vi "arduino_commands_subvi.vi"(0 "Shutter off":bool, 1 "Shutter on":bool, 2 "Go to step":bool, 3 "Constant speed":bool, 4 "Current Step":bool, 5 "Set zero":bool, 6 "wait until completion? (T)":bool=TRUE, 8 "Stop":bool, 9 "Argumento":string="50", 10 "Número de motor":string="1", 11 "Directorio scripts ArduinoStepper.py":path=path "C:/Users/franjas/Documents/rutinas-calibracion-slm") -> (7 "Salida termianl":string[](array[string]))   [LabVIEW 2013]
uses:
  <vilib>/regexp/Match Regular Expression.xnode
panel:
  in  "Stop Button":bool
  out "Terminal output":string
  in  "Set speed":bool
  in  "Comando":string
  out "Comando que está siendo enviado a python":string
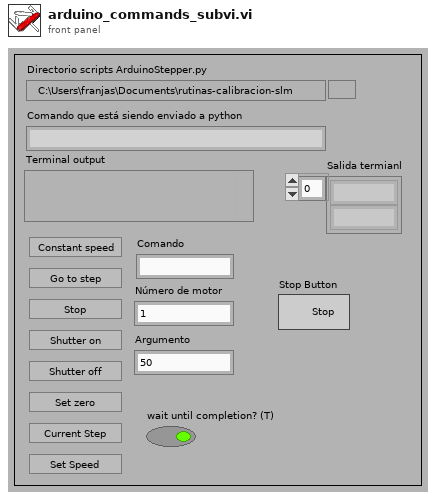
[diagram p1: front panel]
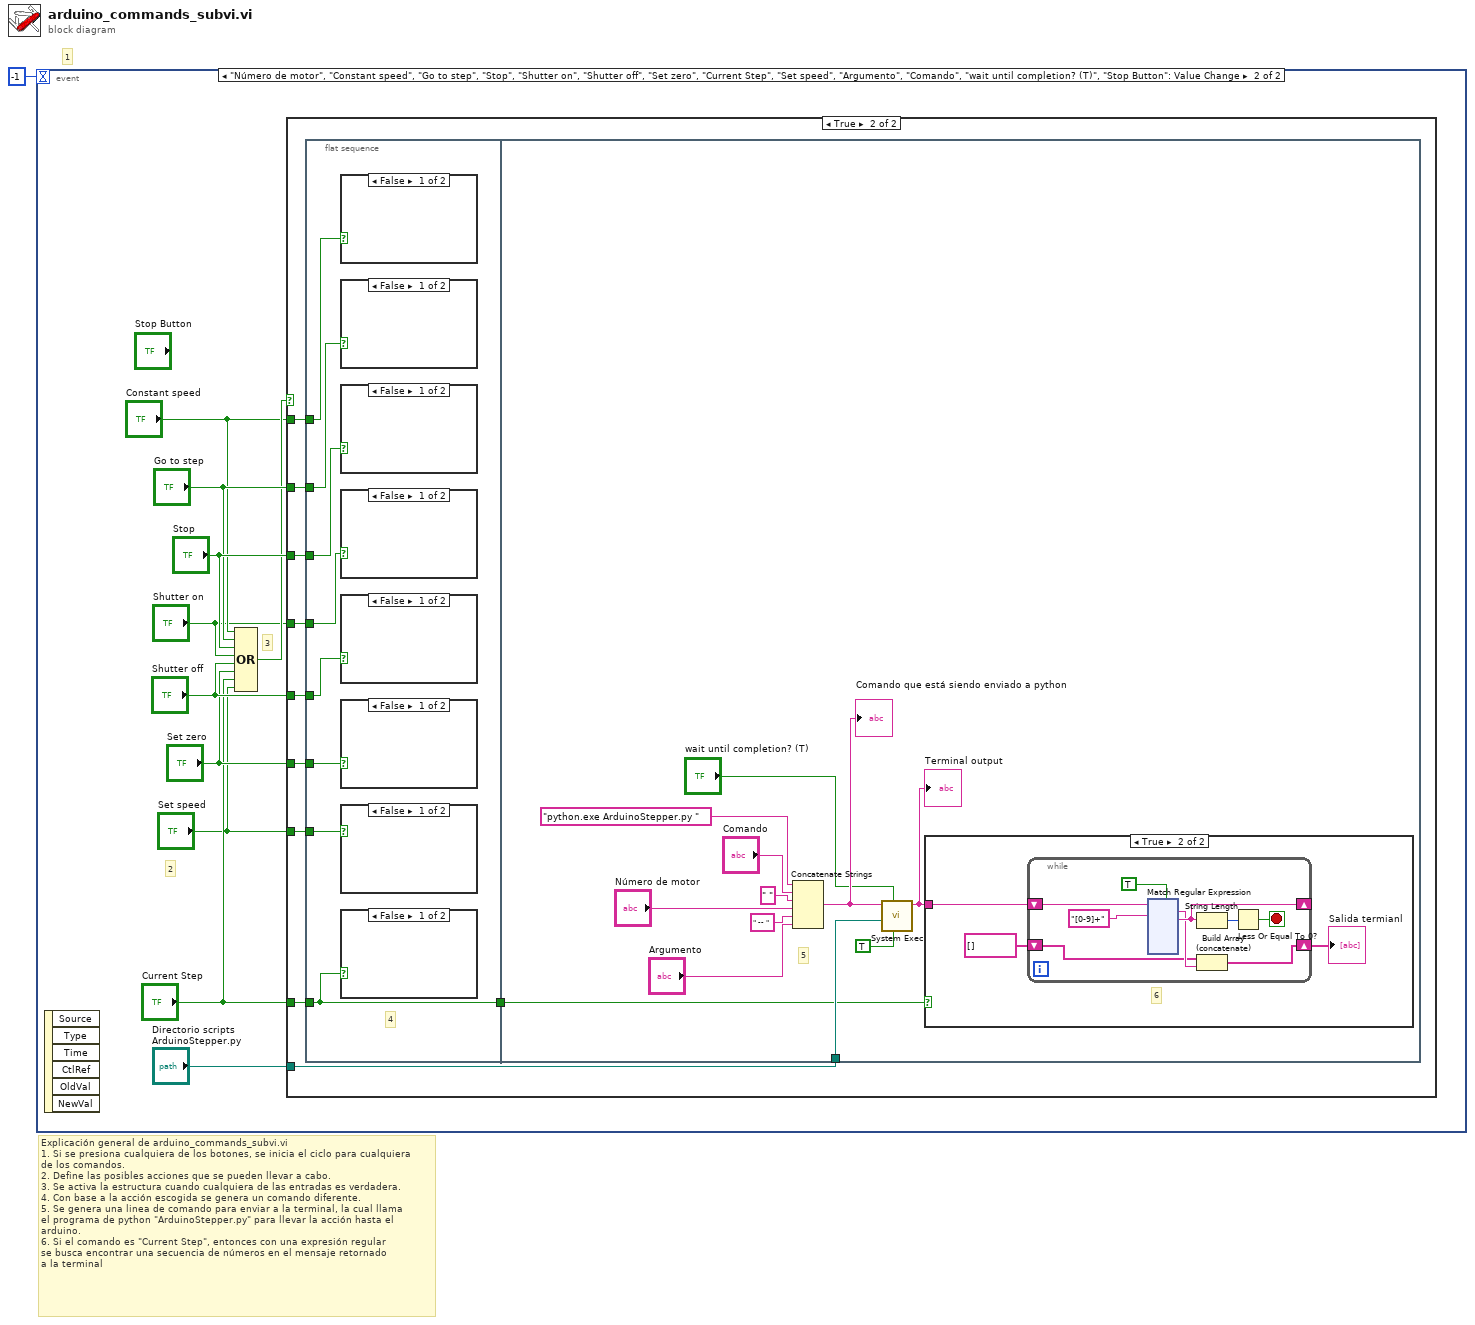
[diagram p0: block diagram]
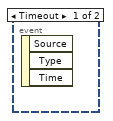
[diagram p2: hidden frame]
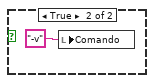
[diagram p4: hidden frame]
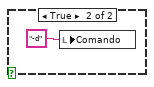
[diagram p5: hidden frame]
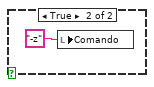
[diagram p6: hidden frame]
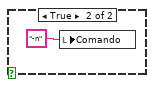
[diagram p7: hidden frame]
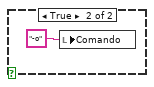
[diagram p8: hidden frame]
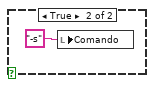
[diagram p9: hidden frame]
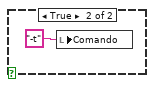
[diagram p10: hidden frame]
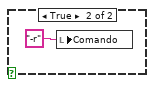
[diagram p11: hidden frame]
diagram:
  # "Explicación general de arduino_commands_subvi.vi\n1. Si se presiona cualquiera de los botones, se inicia el ciclo para cualquiera\nde los comandos.\n2. Define las posibles acciones que se pueden llevar a cabo.\n3. Se activa la estructura cuando cualquiera de las entradas es verdadera.\n4. Con base a la acción escogida se genera un comando diferente.\n5. Se genera una linea de comando para enviar a la terminal, la cual llama\nel programa de python \"ArduinoStepper.py\" para llevar la acción hasta el\narduino.\n6. Si el comando es \"Current Step\", entonces con una expresión regular\nse busca encontrar una secuencia de números en el mensaje retornado\na la terminal"
  # "1"
  n1 = event shown="[1] \"Número de motor\", \"Constant speed\", \"Go to step\", \"Stop\", \"Shutter on\", \"Shutter off\", \"Set zero\", \"Current Step\", \"Set speed\", \"Argumento\", \"Comando\", \"wait until completion? (T)\", \"Stop Button\": Value Change" {
    selector: _ -> [_ _]
    dyn-events: _ -> [_ _]
    timeout: -1 -> [_ _]
    event Timeout {
      n2 = event-data() -> ()  [unwired: 1 in, 3 out]
    }
    event "Número de motor", "Constant speed", "Go to step", "Stop", "Shutter on", "Shutter off", "Set zero", "Current Step", "Set speed", "Argumento", "Comando", "wait until completion? (T)", "Stop Button": Value Change {
      # "3"
      # "2"
      n3 = event-data() -> ()  [unwired: 1 in, 6 out]
      n4 = Compound Arithmetic op=OR("Constant speed", "Go to step", "Stop", "Shutter on", "Shutter off", "Set zero", "Current Step", "Set speed") -> (w8:bool)
      n5 = case shown="True" w8 {
        tunnel: "Directorio scripts ArduinoStepper.py" -> [_ w19]
        tunnel: "Constant speed" -> [_ w21]
        tunnel: "Go to step" -> [_ w18]
        tunnel: "Stop" -> [_ w20]
        tunnel: "Shutter on" -> [_ w17]
        tunnel: "Shutter off" -> [_ w16]
        tunnel: "Set zero" -> [_ w15]
        tunnel: "Current Step" -> [_ w14]
        tunnel: "Set speed" -> [_ w12]
        frame False {
        }
        frame True {
          n6 = flat-sequence {
            tunnel: w21 -> [w29]
            tunnel: w18 -> [w28]
            tunnel: w20 -> [w27]
            tunnel: w17 -> [w26]
            tunnel: w16 -> [w25]
            tunnel: w15 -> [w24]
            tunnel: w14 -> [w23]
            tunnel: [w23] -> w13
            tunnel: w12 -> [w22]
            tunnel: w19 -> [w49]
            tunnel: w13 -> [w40]
            frame #0 {
              # "4"
              n7 = case shown="False" w29 {
                frame False {
                }
                frame True {
                  n8 = local write "Comando"("-r" ("Comando")) -> ()
                }
              }
              n9 = case shown="False" w28 {
                frame False {
                }
                frame True {
                  n10 = local write "Comando"("-t" ("Comando")) -> ()
                }
              }
              n11 = case shown="False" w27 {
                frame False {
                }
                frame True {
                  n12 = local write "Comando"("-s" ("Comando")) -> ()
                }
              }
              n13 = case shown="False" w26 {
                frame False {
                }
                frame True {
                  n14 = local write "Comando"("-o" ("Comando")) -> ()
                }
              }
              n15 = case shown="False" w25 {
                frame False {
                }
                frame True {
                  n16 = local write "Comando"("-n" ("Comando")) -> ()
                }
              }
              n17 = case shown="False" w24 {
                frame False {
                }
                frame True {
                  n18 = local write "Comando"("-z" ("Comando")) -> ()
                }
              }
              n19 = case shown="False" w22 {
                frame False {
                }
                frame True {
                  n20 = local write "Comando"("-v" ("Comando")) -> ()
                }
              }
              n21 = case shown="False" w23 {
                frame False {
                }
                frame True {
                  n22 = local write "Comando"("-d" ("Comando")) -> ()
                }
              }
            }
            frame #1 {
              # "5"
              n23 = Concatenate Strings("python.exe ArduinoStepper.py ", "Comando", " " ("string"), "Número de motor", " -- ", "Argumento") -> (w45:string)
              "Comando que está siendo enviado a python" <- w45
              n24 = call <vilib>:"System Exec.vi"("run minimized? (F)"=TRUE, "wait until completion? (T)"="wait until completion? (T)", "working directory"=w49, "command line"=w45) -> ("standard output"=w41:string)  [unwired: 4 in, 3 out]
              "Terminal output" <- w41
              n25 = case shown="True" w40 {
                tunnel: w41 -> [_ w52]
                frame False {
                }
                frame True {
                  # "6"
                  n26 = while {
                    shift-right: [w59] -> _
                    shift-left: w52 -> [w60]
                    shift-right: [w56] -> w51
                    shift-left: string[] [] -> [w54]
                    stop <- w57 stop-if-true
                    n27 = xnode "Match Regular Expression"("input string"=w60, "regular expression"="[0-9]+", "multiline? (F)"=TRUE) -> ("whole match"=w55:string, "after match"=w59:string)  [unwired: 3 in, 5 out]
                    n28 = String Length(string=w59) -> (length=w58:i32)
                    n29 = Build Array (concatenate)(w54, w55) -> (w56:string[])
                    n30 = Less Or Equal To 0?(x=w58) -> (x <= 0?=w57:bool)
                  }
                  "Salida termianl" <- w51
                }
              }
            }
          }
        }
      }
    }
  }
